vi "Configure Channel (Voltage).vi"(4 "Power Line Cycles (0)":i32, 5 "Current Range:\n0=1uA\n1=10uA\n2=100uA\n3=1mA\n4=10mA\n5=120mA":i32=5, 6 "Triggered Level (1.0 V)":dbl=1.0, 7 "Voltage Range (0: 2 Volts)":u16(ring) items=["2 Volts", "20 Volts"], 8 "error in (no error)":errorcluster, 9 "Output Level (1.0 V)":dbl=1.0, 10 "Channel (1: Channel 1)":u16(ring)=1 items=["Channel 1"=1, "Channel 2"=2, "Channel 3"=3], 11 "VISA resource name":refnum<visa-resource-name>) -> (0 "error out":errorcluster, 3 "VISA resource name out":refnum<visa-resource-name>)   [LabVIEW 2018, in "Agilent U2722.lvlib"]
doc: "Configures the channel to output in source voltage mode."
uses:
  Agilent U2722.lvlib
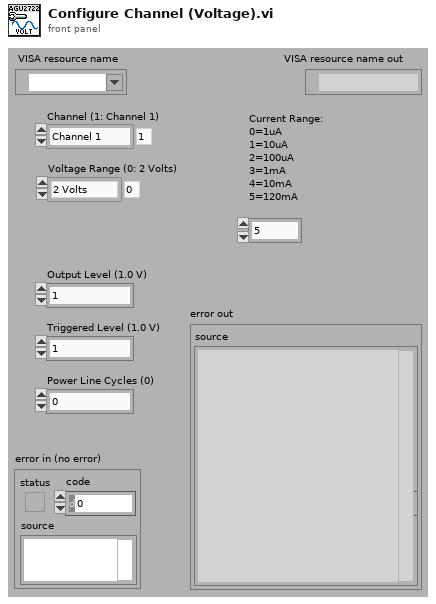
[diagram p1: front panel]
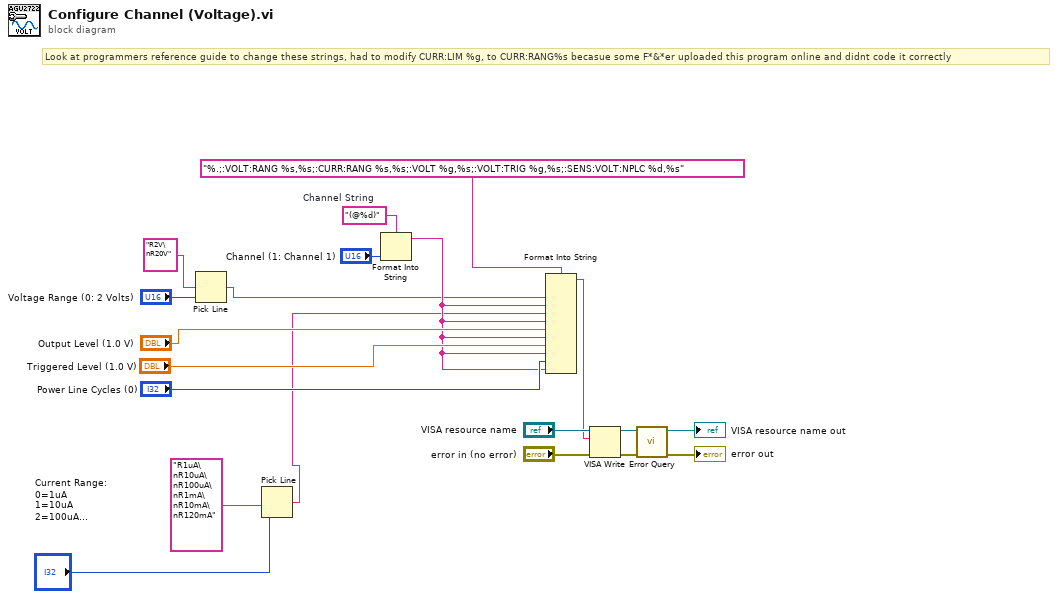
[diagram p0: block diagram]
diagram:
  w13 = "(@%d)"  # Channel String
  # "Look at programmers reference guide to change these strings, had to modify CURR:LIM %g, to CURR:RANG%s becasue some F*&*er uploaded this program online and didnt code it correctly"
  n1 = Pick Line(multi-line string="R2V\nR20V", line index="Voltage Range (0: 2 Volts)") -> (output string=w5:string)  [unwired: 1 in]
  n2 = Pick Line(multi-line string="R1uA\nR10uA\nR100uA\nR1mA\nR10mA\nR120mA", line index="Current Range:\n0=1uA\n1=10uA\n2=100uA\n3=1mA\n4=10mA\n5=120mA") -> (output string=w3:string)  [unwired: 1 in]
  n3 = Format Into String(format string=w13, "Channel (1: Channel 1)") -> (resulting string=w9:string)  [unwired: 2 in, 1 out]
  n4 = Format Into String(format string="%.;:VOLT:RANG %s,%s;:CURR:RANG %s,%s;:VOLT %g,%s;:VOLT:TRIG %g,%s;:SENS:VOLT:NPLC %d,%s", w5, w9, w3, w9, "Output Level (1.0 V)", w9, "Triggered Level (1.0 V)", w9, "Power Line Cycles (0)", w9) -> (resulting string=w8:string)  [unwired: 2 in, 1 out]
  n5 = VISA Write(VISA resource name="VISA resource name", write buffer=w8, error in (no error)="error in (no error)") -> (VISA resource name out=w16:refnum<visa-resource-name>, error out=w15:errorcluster)  [unwired: 1 out]
  n6 = call "Error Query.vi"("error in (no error)"=w15, "VISA resource name"=w16) -> ("error out"=→"error out":errorcluster, "VISA resource name out"=→"VISA resource name out":refnum<visa-resource-name>)  [unwired: 6 in, 2 out]
